vi "telemetry_publisher.vi"() -> ()   [LabVIEW 2016]
uses:
  ts_sallv_exa/DataTypes/LoopTime_ms.ctl
  ts_sallv_exa/DataTypes/Timestamp.ctl
  ts_sallv_exa/SALLV_EXA.lvlib
panel:
  out "Fake Timeloop":T1
  out "Timestamp":string
  out "Stop":bool=TRUE
  in  "stop":bool
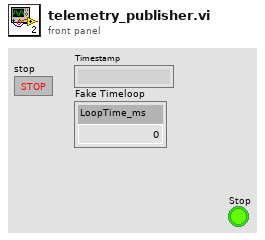
[diagram p1: front panel]
types:
  T1 = typedef "SALLV_EXA.lvlib/LoopTime_ms.ctl" = cluster{"LoopTime_ms":dbl}
  T2 = typedef "SALLV_EXA.lvlib/Timestamp.ctl" = cluster{"Timestamp":string}
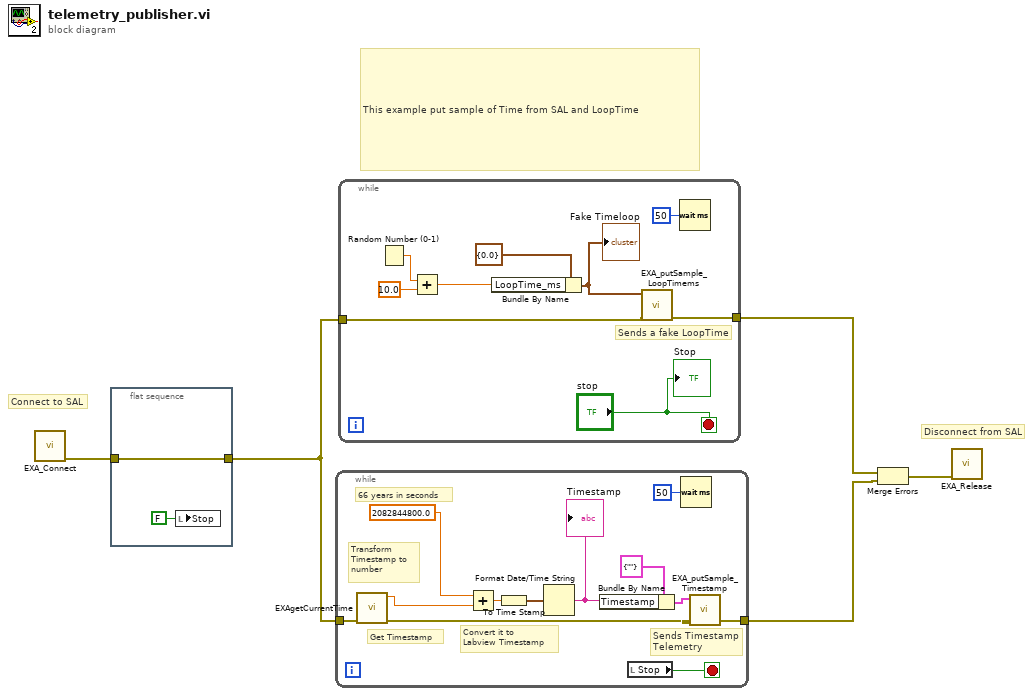
[diagram p0: block diagram]
diagram:
  # "Disconnect from SAL"
  # "Connect to SAL"
  # "This example put sample of Time from SAL and LoopTime"
  n1 = call "EXA_Connect.vi"() -> ("error out"=w3:errorcluster)  [unwired: 10 in, 1 out]
  n2 = flat-sequence {
    tunnel: [w7] -> w2
    tunnel: w3 -> [w7]
    frame #0 {
      n3 = local write "Stop"(FALSE ("Stop")) -> ()
    }
  }
  n4 = while {
    tunnel: w2 -> [w16]
    tunnel: [w17] -> w1
    stop <- w19 stop-if-true
    # "66 years in seconds"
    # "Convert it to \nLabview Timestamp"
    # "Transform\nTimestamp to \nnumber"
    # "Get Timestamp"
    # "Sends Timestamp \nTelemetry"
    n5 = call "EXAgetCurrentTime.vi"("error in (no error)"=w16) -> ("error out"=w15:errorcluster, "function return"=w9:dbl)  [unwired: 9 in]
    n6 = Add(x=2082844800.0, y=w9) -> (x+y=w10:dbl)
    n7 = To Time Stamp(1:w10) -> (0:w13:timestamp)
    n8 = Format Date/Time String(seconds (now)=w13) -> (date/time string=w12:string)  [unwired: 2 in]
    "Timestamp" <- w12
    n9 = Bundle By Name(cluster=T2 {"Timestamp"=""} ("Timestamp_Ctl"), "Timestamp"=w12) -> (w11:T2)
    n10 = local read "Stop"() -> (w19:bool)
    n11 = Wait (ms)(milliseconds to wait=u32 50) -> ()  [unwired: 1 out]
    n12 = call "EXA_putSample_Timestamp.vi"("error in (no error)"=w15, "Timestamp_Ctl"=w11) -> ("error out"=w17:errorcluster)  [unwired: 7 in, 2 out]
  }
  n13 = while {
    tunnel: w2 -> [w26]
    tunnel: [w25] -> w4
    stop <- "stop" stop-if-true
    # "Sends a fake LoopTime"
    n14 = Random Number (0-1)() -> (number: 0 to 1=w22:dbl)
    n15 = Add(x=w22, y=10.0) -> (x+y=w21:dbl)
    n16 = Bundle By Name(cluster=T1 {"LoopTime_ms"=0.0} ("LoopTime_ms_Ctl"), "LoopTime_ms"=w21) -> (w23:T1)
    "Fake Timeloop" <- w23
    n17 = call "EXA_putSample_LoopTimems.vi"("error in (no error)"=w26, "LoopTime_ms_Ctl"=w23) -> ("error out"=w25:errorcluster)  [unwired: 7 in, 2 out]
    n18 = Wait (ms)(milliseconds to wait=u32 50) -> ()  [unwired: 1 out]
    "Stop" <- "stop"
  }
  n19 = Merge Errors(w4, w1) -> (w5:errorcluster)
  n20 = call "EXA_Release.vi"("error in (no error)"=w5) -> ()  [unwired: 9 in, 2 out]
